vi "SR430_set_discriminator_slope.vi"(0 "address":T1, 2 "discriminatorSlope":bool, 5 "error in (no error)":errorcluster) -> (14 "address out":T1, 19 "error out":errorcluster)   [LabVIEW 2015, in "SR430Driver.lvlib"]
doc: "Sets the discriminator slope. \n\nCopyright (C)\nGesellschaft für Schwerionenforschung, GSI\nPlanckstr. 1\n64291 Darmstadt\nGermany\n\nContact: D.Beck@gsi.de \n\nThis program is free software; you can redistribute it and/or modify it under the terms of the \nGNU General Public License as published by the Free Software Foundation; either version 2 of the license, or (at your option) any later version.\n\nThis program is distributed in the hope that it will be useful, but WITHOUT ANY WARRANTY; without even the implied warranty of MERCHANTABILITY or FITNESS FOR A PARTICULAR PURPOSE. See the GNU General License for more details (http://www.gnu.org).\n\nGesellschaft für Schwerionenforschung, GSI\nPlanckstr. 1, 64291 Darmstadt, Germany\nFor all questions and ideas contact: M.Richter@gsi.de, K.Poppensieker, H.Brand@gsi.de or D.Beck@gsi.de.\nLast update: 11-APR-2002"
uses:
  SR430Driver.lvlib
  SR430_VISA Control.ctl
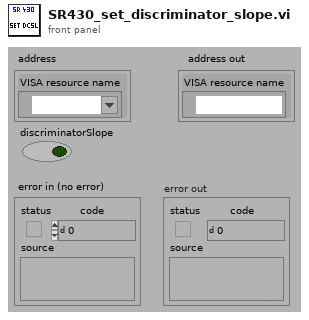
[diagram p1: front panel]
types:
  T1 = typedef "SR430Driver.lvlib/SR430_VISA Control.ctl" = cluster{"VISA resource name":refnum<visa-resource-name>}
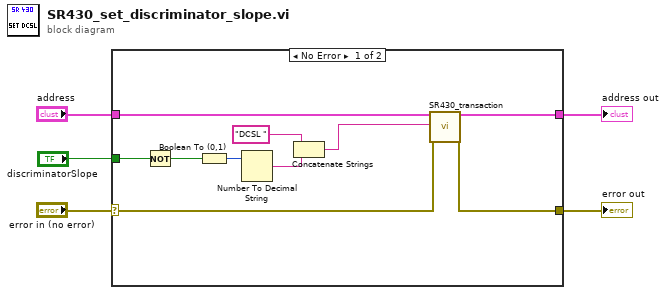
[diagram p0: block diagram]
diagram:
  n1 = case shown="No Error" "error in (no error)" {
    selector: "error in (no error)" -> [w8 w16]
    tunnel: "address" -> [w10 w17]
    tunnel: [w9 w17] -> w4
    tunnel: [w7 w16] -> w3
    tunnel: "discriminatorSlope" -> [w14 _]
    frame No Error {
      n2 = Not(x=w14) -> (.not. x?=w11:bool)
      n3 = Boolean To (0,1)(Boolean=w11) -> (0, 1=w13:i16)
      n4 = Number To Decimal String(number=w13) -> (decimal integer string=w12:string)  [unwired: 1 in]
      n5 = Concatenate Strings("DCSL ", w12) -> (w6:string)
      n6 = call "SR430_transaction.vi"("SR430 VISA Cluster"=w10, "SR430 Command String"=w6, "error in (no error)"=w8) -> ("dup SR430 VISA Cluster"=w9:T1, "error out"=w7:errorcluster)  [unwired: 13 in, 2 out]
    }
    frame Error {
    }
  }
  "address out" <- w4
  "error out" <- w3
